vi "Universal_Ramping.vi"(5 "address string":string, 6 "error in (no error)":errorcluster, 7 "VISA command":string="smua.source.leveli=", 8 "Voltage Step (V)":dbl=0.01 caption="Step Value", 9 "Final Voltage (V)":dbl=0.1 caption="Final Value", 10 "Initial Voltage (V)":dbl caption="Initial Value", 11 "VISA resource name":refnum<visa-resource-name>) -> (0 "error out":errorcluster, 2 "Actual Voltage (V)":dbl caption="Actual Value" step=0.1, 3 "Ready":bool)   [LabVIEW 2015]
panel:
  out "Visa Command":string
  out "Increase/Decrease":string
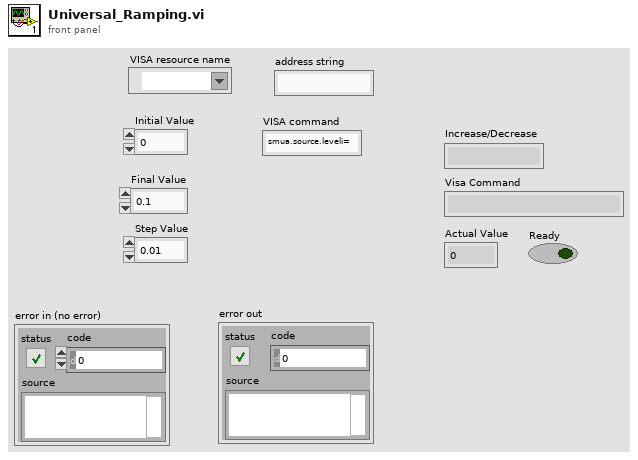
[diagram p1: front panel]
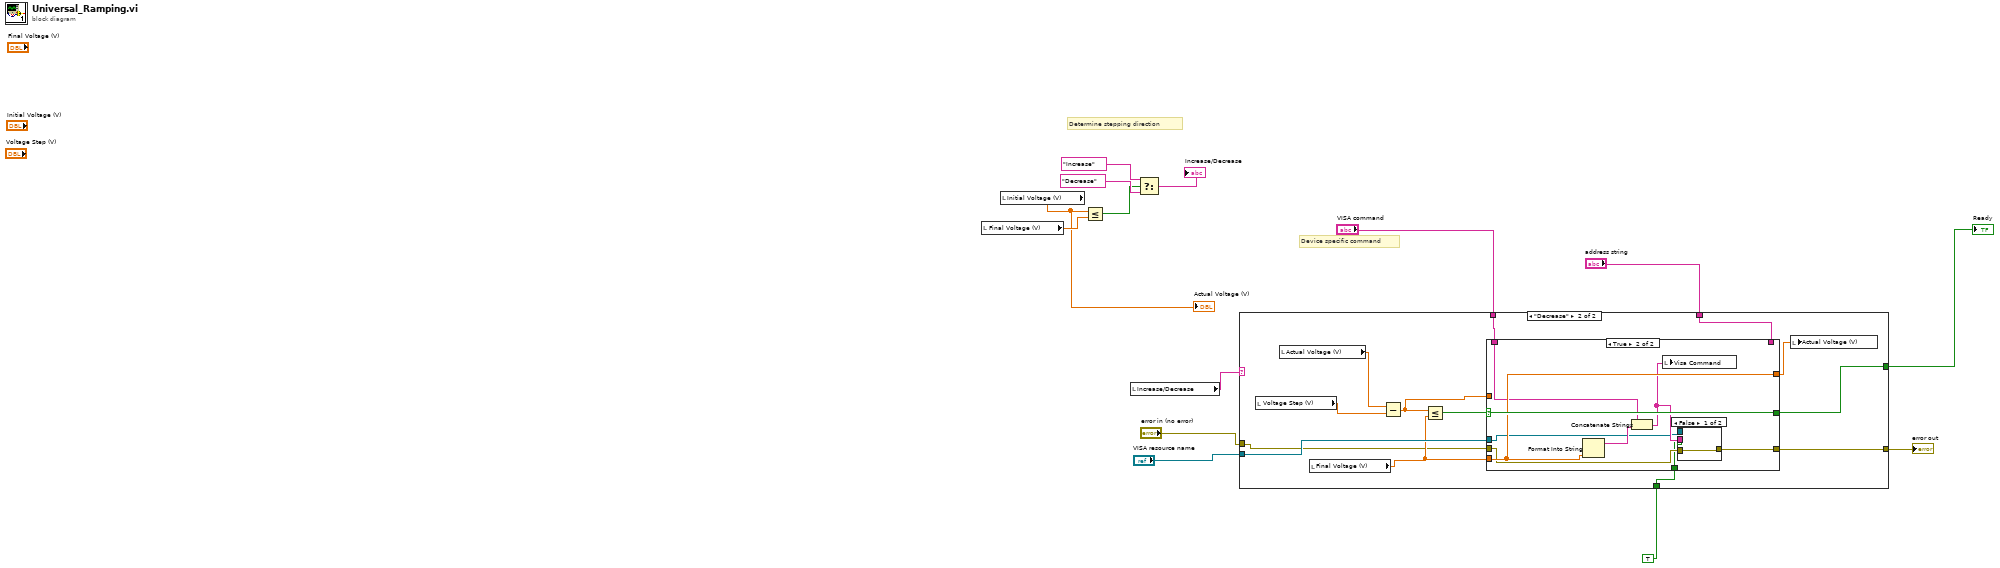
[diagram p0: block diagram]
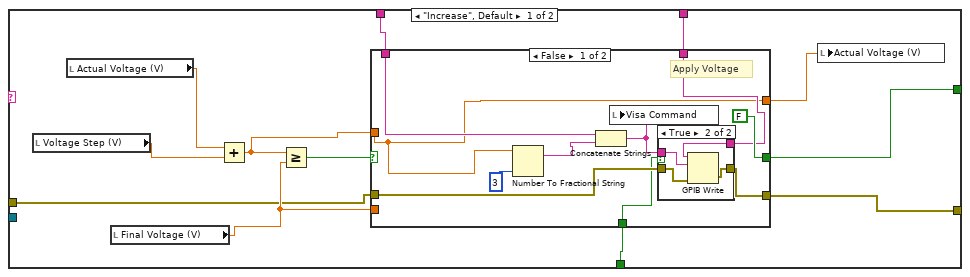
[diagram p2: hidden frame]
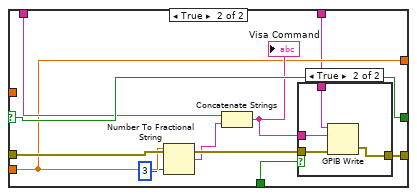
[diagram p4: hidden frame]
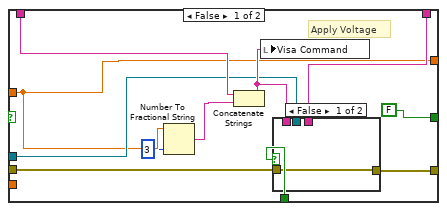
[diagram p6: hidden frame]
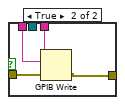
[diagram p7: hidden frame]
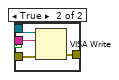
[diagram p8: hidden frame]
diagram:
  # "Device specific command"
  # "Determine stepping direction"
  n1 = local read "Final Voltage (V)"() -> (w14:dbl)
  n2 = local read "Initial Voltage (V)"() -> (w2:dbl)
  "Actual Voltage (V)" <- w2
  n3 = Less Or Equal?(x=w2, y=w14) -> (x <= y?=w10:bool)
  n4 = local read "Increase/Decrease"() -> (w6:string)
  n5 = Select(t="Increase", s=w10, f="Decrease") -> (s? t:f=→"Increase/Decrease":string)
  n6 = case shown="\"Decrease\"" w6 {
    tunnel: [w24 w66] -> w5
    tunnel: "VISA resource name" -> [_ w67]
    tunnel: "VISA command" -> [w19 w61]
    tunnel: "error in (no error)" -> [w18 w59]
    tunnel: [w17 w60] -> w3
    tunnel: TRUE -> [w16 w58]
    tunnel: "address string" -> [w15 w57]
    frame "Increase", Default {
      n7 = local read "Voltage Step (V)"() -> (w23:dbl)
      n8 = local read "Actual Voltage (V)"() -> (w22:dbl)
      n9 = local read "Final Voltage (V)"() -> (w20:dbl)
      n10 = Add(x=w22, y=w23) -> (x+y=w26:dbl)
      n11 = Greater Or Equal?(x=w26, y=w20) -> (x >= y?=w25:bool)
      n12 = case shown="False" w25 {
        selector: w25 -> [_ w51]
        tunnel: [FALSE w51] -> w24
        tunnel: w26 -> [w29 _]
        tunnel: [w29 w45] -> w21
        tunnel: w20 -> [_ w45]
        tunnel: w19 -> [w36 w50]
        tunnel: w18 -> [w35 w48]
        tunnel: [w34 w47] -> w17
        tunnel: w16 -> [w32 w46]
        tunnel: w15 -> [w30 w42]
        frame False {
          # "Apply Voltage"
          n13 = Number To Fractional String(number=w29, precision (6)=i16 3) -> (F-format string=w28:string)  [unwired: 2 in]
          n14 = Concatenate Strings(w36, w28) -> (w33:string)
          n15 = local write "Visa Command"(w33) -> ()
          n16 = case shown="True" w32 {
            tunnel: w35 -> [w37 w39]
            tunnel: [w37 w38] -> w34
            tunnel: w33 -> [_ w40]
            tunnel: w30 -> [_ w41]
            frame False {
            }
            frame True {
              n17 = GPIB Write(0:w41, 1:w40, 3:w39) -> (6:w38:errorcluster)  [unwired: 2 in, 1 out]
            }
          }
        }
        frame True {
          n18 = Number To Fractional String(number=w45, precision (6)=i16 3) -> (F-format string=w44:string)  [unwired: 2 in]
          n19 = Concatenate Strings(w50, w44) -> (w49:string)
          "Visa Command" <- w49
          n20 = case shown="True" w46 {
            tunnel: w49 -> [_ w54]
            tunnel: w48 -> [w52 w55]
            tunnel: [w52 w56] -> w47
            tunnel: w42 -> [_ w53]
            frame False {
            }
            frame True {
              n21 = GPIB Write(0:w53, 1:w54, 3:w55) -> (6:w56:errorcluster)  [unwired: 2 in, 1 out]
            }
          }
        }
      }
      n22 = local write "Actual Voltage (V)"(w21) -> ()
    }
    frame "Decrease" {
      n23 = local read "Voltage Step (V)"() -> (w65:dbl)
      n24 = local read "Actual Voltage (V)"() -> (w64:dbl)
      n25 = local read "Final Voltage (V)"() -> (w62:dbl)
      n26 = Subtract(x=w64, y=w65) -> (x-y=w69:dbl)
      n27 = Less Or Equal?(x=w69, y=w62) -> (x <= y?=w68:bool)
      n28 = case shown="True" w68 {
        selector: w68 -> [_ w94]
        tunnel: [FALSE w94] -> w66
        tunnel: w69 -> [w72 _]
        tunnel: w67 -> [w77 w89]
        tunnel: [w72 w92] -> w63
        tunnel: w62 -> [_ w92]
        tunnel: w61 -> [w79 w91]
        tunnel: [w76 w87] -> w60
        tunnel: w59 -> [w75 w88]
        tunnel: w58 -> [w74 w86]
        tunnel: w57 -> [w73 _]
        frame False {
          # "Apply Voltage"
          n29 = Number To Fractional String(number=w72, precision (6)=i16 3) -> (F-format string=w70:string)  [unwired: 2 in]
          n30 = Concatenate Strings(w79, w70) -> (w78:string)
          n31 = local write "Visa Command"(w78) -> ()
          n32 = case shown="False" w74 {
            tunnel: w78 -> [_ w84]
            tunnel: w77 -> [_ _]
            tunnel: [w81 w82] -> w76
            tunnel: w75 -> [w81 w83]
            tunnel: w73 -> [_ w85]
            frame False {
            }
            frame True {
              n33 = GPIB Write(0:w85, 1:w84, 3:w83) -> (6:w82:errorcluster)  [unwired: 2 in, 1 out]
            }
          }
        }
        frame True {
          n34 = Format Into String(w92) -> (resulting string=w93:string)  [unwired: 3 in, 1 out]
          n35 = Concatenate Strings(w91, w93) -> (w90:string)
          n36 = local write "Visa Command"(w90) -> ()
          n37 = case shown="False" w86 {
            tunnel: w90 -> [_ w99]
            tunnel: w89 -> [_ w98]
            tunnel: w88 -> [w95 w97]
            tunnel: [w95 w96] -> w87
            frame False {
            }
            frame True {
              n38 = VISA Write(VISA resource name=w98, write buffer=w99, error in (no error)=w97) -> (error out=w96:errorcluster)  [unwired: 2 out]
            }
          }
        }
      }
      n39 = local write "Actual Voltage (V)"(w63) -> ()
    }
  }
  "Ready" <- w5
  "error out" <- w3
